vi "Process.vi"(8 "error in":errorcluster, 11 "Instrument UI.Framework-Template":refnum<class "Instrument UI.Framework-Template.lvclass">) -> (0 "error out":errorcluster, 3 "Instrument UI.Framework-Template out":refnum<class "Instrument UI.Framework-Template.lvclass">)   [LabVIEW 2019, in "Instrument UI.Framework-Template.lvclass"]
doc: "---------------------------------------------------------------\nJKI State Machine Objects™\nhttp://jki.net/state-machine-objects/\nCopyright (C) 2005-2015, JKI <info@jki.net>\nALL RIGHTS RESERVEDJKI State Machine Objects (SMO) 1.0.0.5\nJKI - JKI\nCopyright (c) 2016, JKI"
uses:
  Instrument UI.Framework-Template.lvclass
  C:/Program Files (x86)/National Instruments/LabVIEW 2019/vi.lib/JKI/JKI SMO/SMO/SMO.lvclass
  C:/Program Files (x86)/National Instruments/LabVIEW 2019/user.lib/LevyLab/Instrument Framework/Instrument UI/Instrument UI.lvclass
  C:/Program Files (x86)/National Instruments/LabVIEW 2019/vi.lib/JKI/JKI SMO/SMO.UI/SMO.UI.lvclass
  Instrument.Framework-Template/Typedefs/Instrument.Framework-Template.getAll--Cluster.ctl
  Instrument.Framework-Template/Instrument.Framework-Template.lvclass
  C:/Program Files (x86)/National Instruments/LabVIEW 2019/user.lib/LevyLab/Instrument Framework/Instrument/Instrument.lvclass
  Instrument UI.Framework-Template.UI--Cluster.ctl
  Instrument.Framework-Template/Typedefs/Instrument.Framework-Template.Configuration--Cluster.ctl
  <userlib>/LevyLab/Configuration/Configuration.lvclass
  <userlib>/LevyLab/Instrument Framework/Instrument UI/Instrument UI.lvclass/Instrument UI.ctl
  <vilib>/JKI/JKI SMO/SMO/SMO.lvclass/SMO.ctl
  <userlib>/LevyLab/Configuration/Configuration.lvclass/Configuration.ctl
  2c224a34-a253-4174-b18d-44043a318d1a.vi
  <vilib>/JKI/JKI SMO/SMO/Private/ReftoDVR--SMO.vi
  2c224a34-a253-4174-b18d-44043a318d1a.vi/26bc7fe7-399c-42c0-9e9a-60ca208975aa.vi
  2c224a34-a253-4174-b18d-44043a318d1a.vi/9995e869-8f6f-46da-9c29-74663bf4c27c.vi
  <vilib>/Utility/Data Type/Get Type Information.vi
  <vilib>/JDP Science/JSONtext/JSON text to Variant.vi
  <userlib>/LevyLab/Instrument Framework/Instrument/Instrument.lvclass
  <vilib>/JDP Science/JSONtext/LVClass Serializer/JSONtext LVClass Serializer.lvclass
  <userlib>/LevyLab/Instrument Framework/Instrument UI/Instrument UI.lvclass
  <vilib>/JKI/JKI SMO/SMO/SMO.lvclass
  <vilib>/JKI/JKI SMO/SMO.UI/SMO.UI.lvclass
  <userlib>/LevyLab/Debug/Debug.lvlib
panel:
  out "State History":string
  in  "Parameter 2":string
  out "Numeric":u32
  in  "Set Parameter":bool
  in  "Parameter":dbl
  in  "STOP":bool
  out "SMO string":string
  out "SMO Boolean":bool
  out "Logger SMO":dbl
  out "Levy 1":dbl
  # "#todo\nmake UI here. maybe include a nice picture of the hardware?"
  # "#todo\nadd buttons to do stuff (e.g., change a setting)\nButtons should trigger an event"
  # "#todo\nresize this box if you want your UI to be different size"
  # "SMO UI Template"
  # "For instructions on how to use the JKI State Machine Objects, examples and video tutorials, visit:\nhttp://jki.net/state-machine-objects/\n\nJKI State Machine Objects™\nhttp://jki.net/state-machine-objects/\nCopyright (C) 2005-2015, JKI <info@jki.net>\nALL RIGHTS RESERVED"
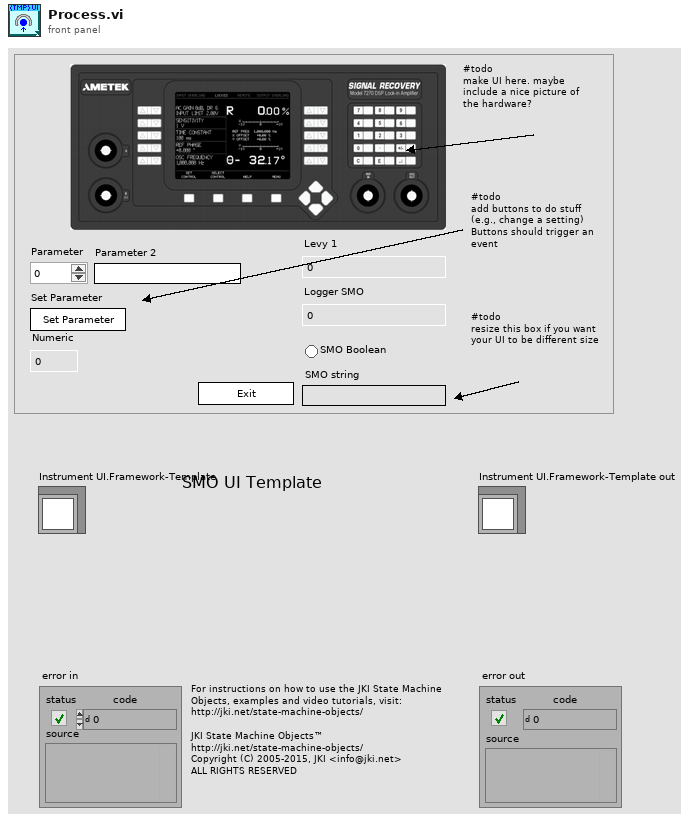
[diagram p1: front panel]
types:
  T1 = enum32{"invalid app kind", "Development System", "Run Time System", "Student Edition", "Embedded LabVIEW", "Evaluation", "Custom"}
  T2 = enum32{"Invalid", "Standard", "Closed", "Hidden", "Minimized", "Maximized"}
  T3 = typedef "Instrument.Framework-Template.lvclass/Instrument.Framework-Template.Configuration--Cluster.ctl" = cluster{"Example Setting 1":dbl, "Example Setting 2":dbl, "Example Setting 3":string}
  T4 = typedef "Instrument.Framework-Template.lvclass/Instrument.Framework-Template.getAll--Cluster.ctl" = cluster{"Levy 1":dbl, "Logger SMO":dbl, "SMO Boolean":bool, "SMO String":string}
  T5 = typedef "Instrument UI.Framework-Template.lvclass/Instrument UI.Framework-Template.UI--Cluster.ctl" = cluster{"Parameter":dbl, "Parameter 2":string}
  T6 = cluster{"Core":cluster{"Current VI Reference":refnum<vi>, "Close Panel on Exit?":bool, "Last Error":cluster{"error":errorcluster, "previous state":string, "remaining states":string}, "Shutdown?":bool}, "Instrument UI":refnum<class "Instrument UI.Framework-Template.lvclass">, "Instrument":refnum<class "Instrument.Framework-Template.lvclass">, "Configuration":refnum<class "Configuration.lvclass">, "Config Cluster":T3, "getAll":T4, "UI Cluster":T5, "UI Behavior":string, "wait":u32}
  T7 = cluster{"Current VI Reference":refnum<vi>, "Close Panel on Exit?":bool, "Last Error":cluster{"error":errorcluster, "previous state":string, "remaining states":string}, "Shutdown?":bool}
  T8 = typedef "Debug.lvlib/Attribute.Debug.lvclass/DebugBehavior.ctl" = enum16{"Normal", "Debug"}
  T9 = typedef "smo.lvlib/SMO.lvclass/Protected Events.ctl" = cluster{"StopProcesses":refnum<user-event>, "AbortProcesses":refnum<user-event>, "Config Changed":refnum<user-event>, "Dependency":refnum<user-event>}
  T10 = typedef "Instrument.lvlib/Instrument.lvclass/PublicEvents--Cluster.ctl" = cluster{"MessageFromProcess":refnum<user-event>}
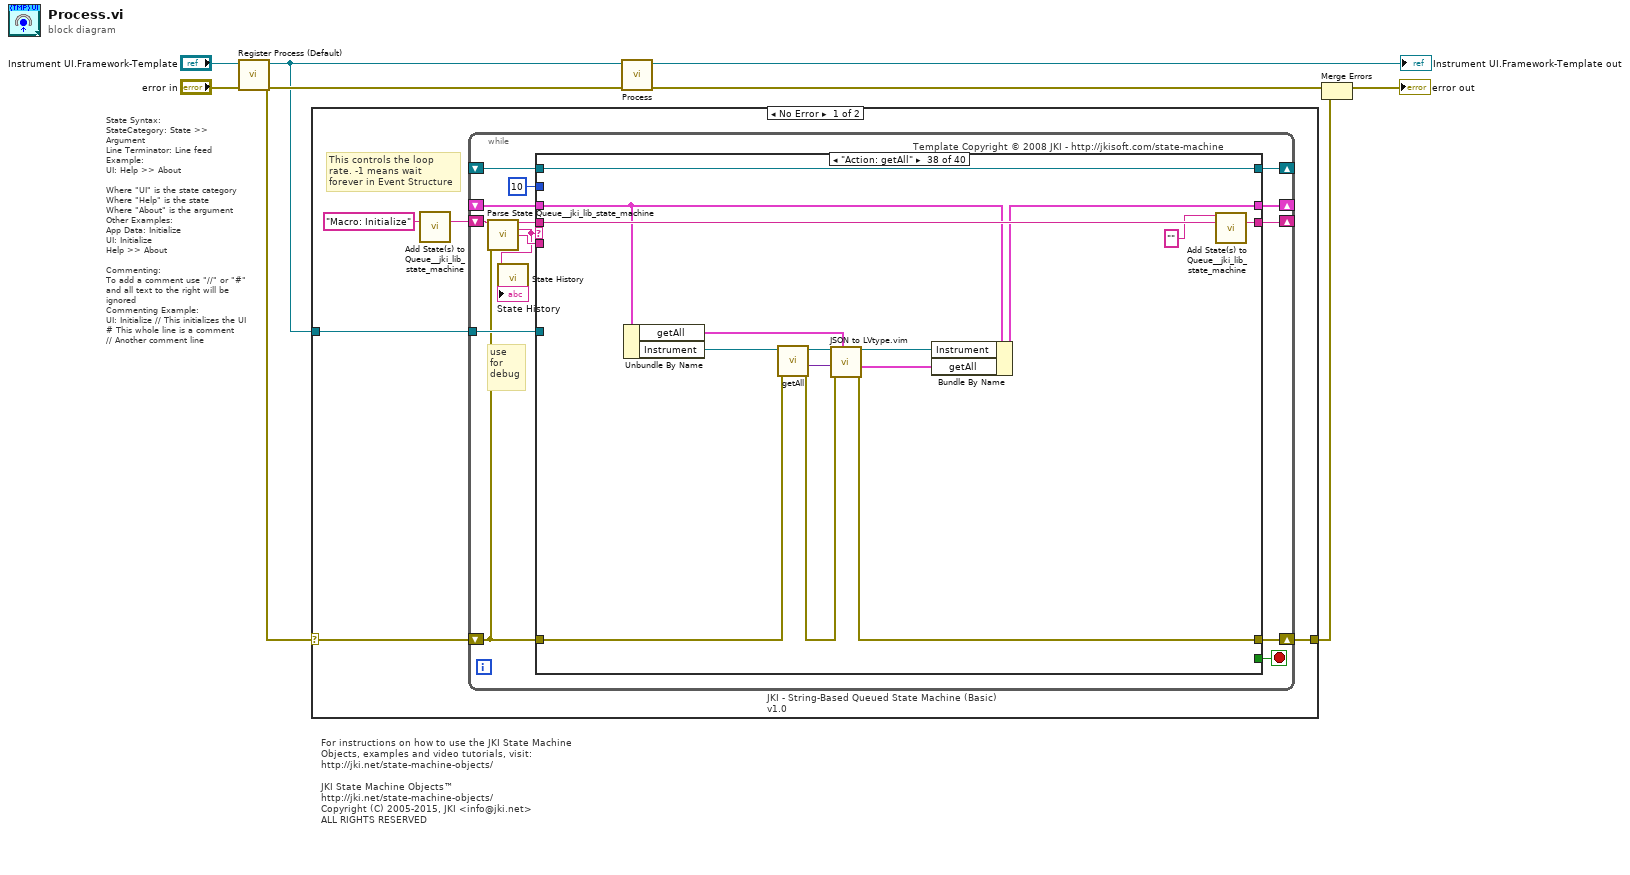
[diagram p0: block diagram]
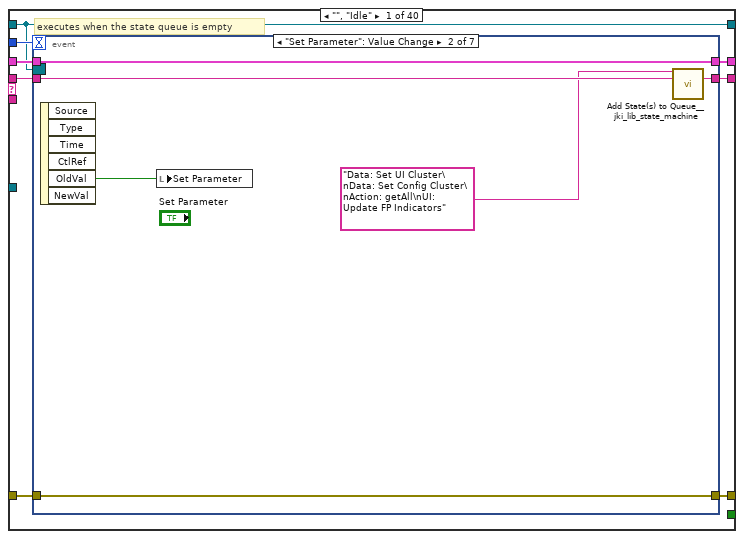
[diagram p2: hidden frame]
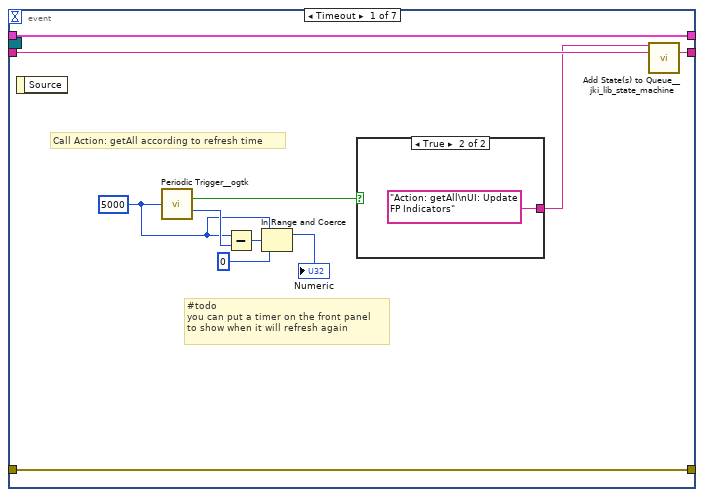
[diagram p3: hidden frame]
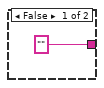
[diagram p4: hidden frame]
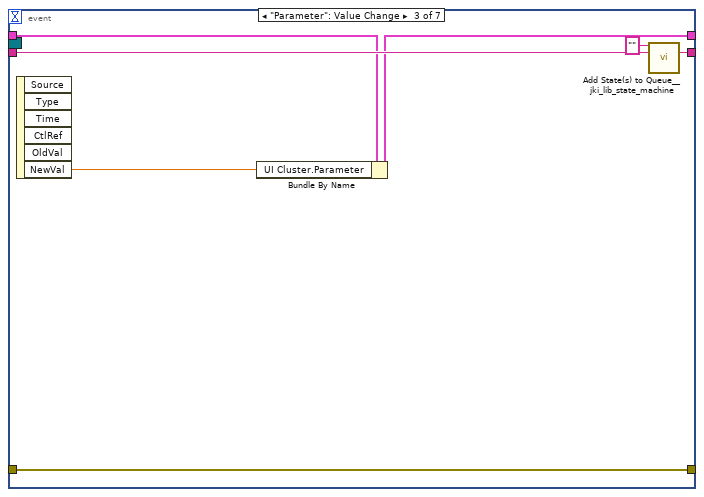
[diagram p5: hidden frame]
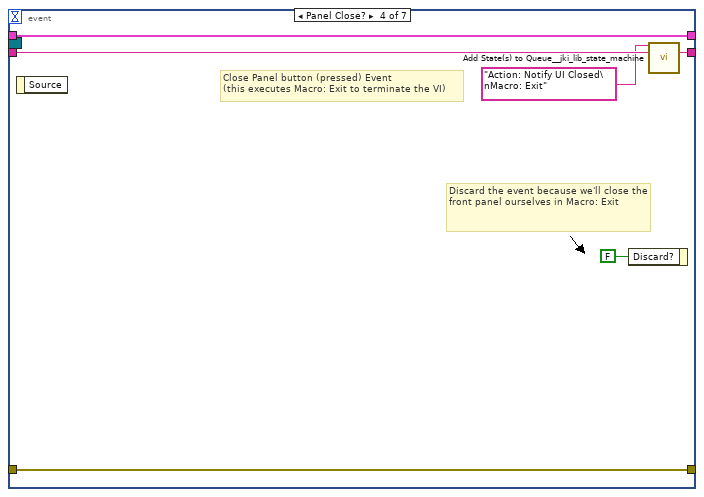
[diagram p6: hidden frame]
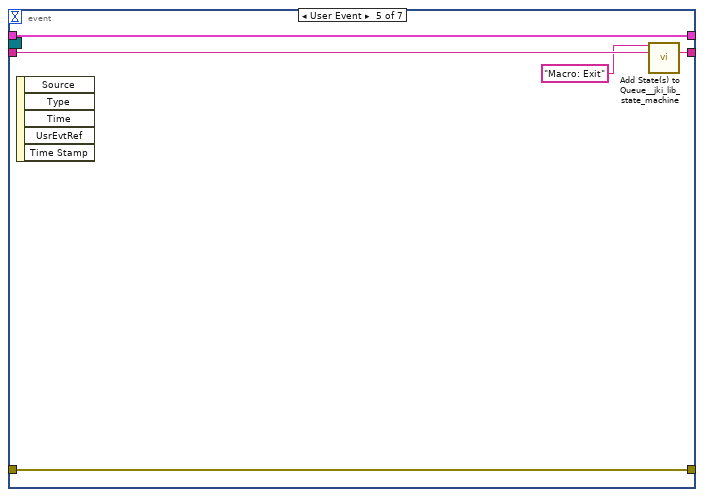
[diagram p7: hidden frame]
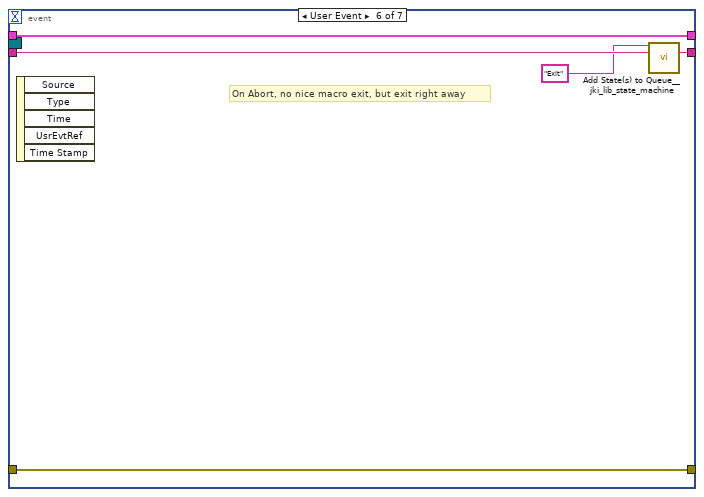
[diagram p8: hidden frame]
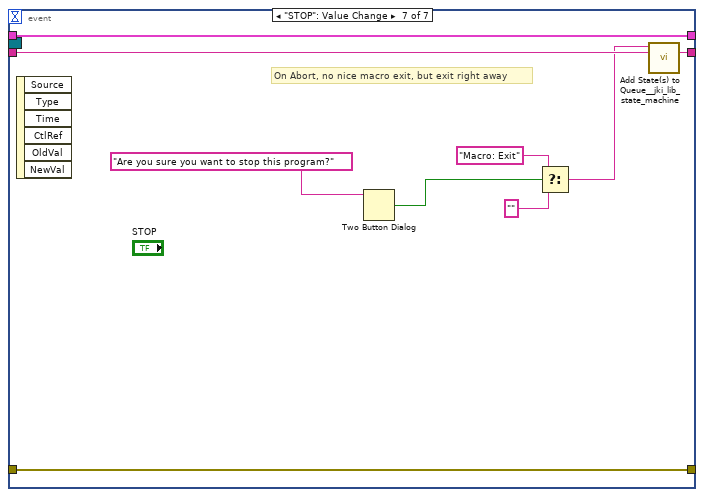
[diagram p9: hidden frame]
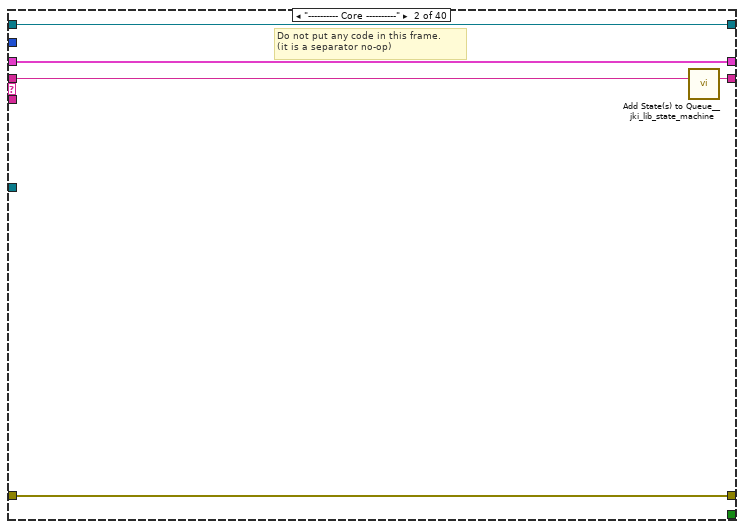
[diagram p10: hidden frame]
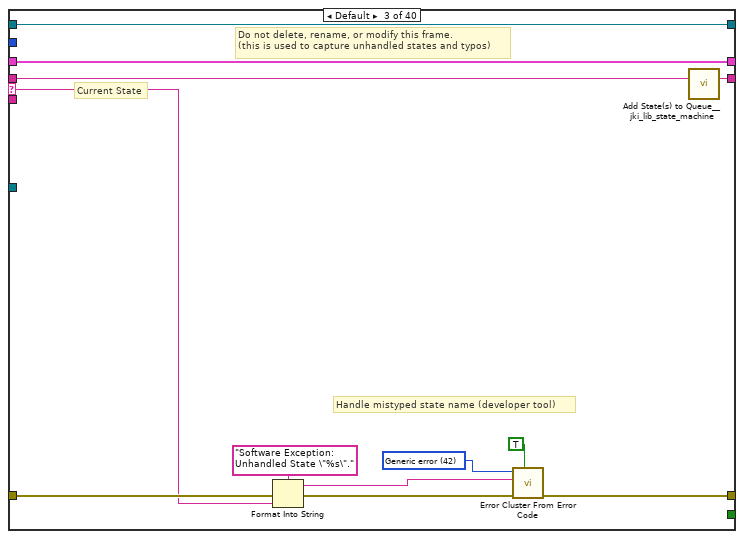
[diagram p11: hidden frame]
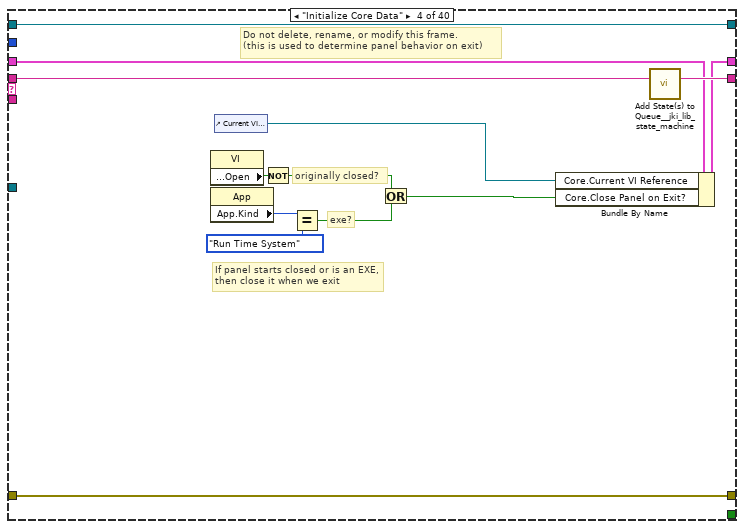
[diagram p12: hidden frame]
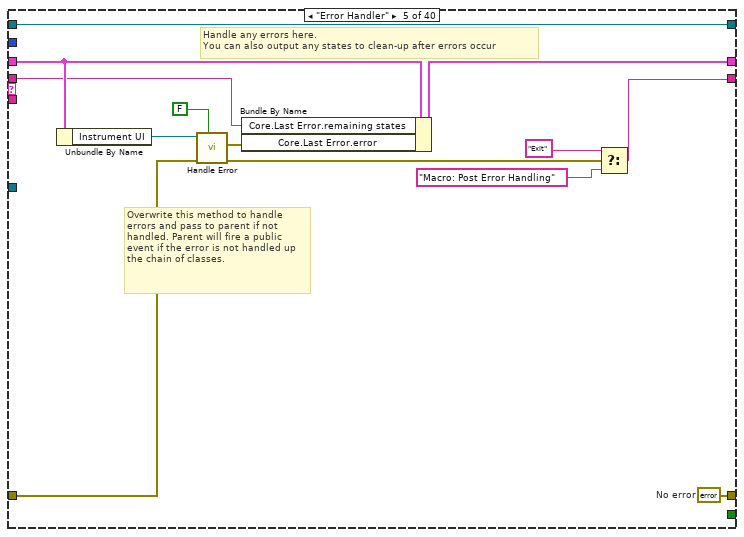
[diagram p13: hidden frame]
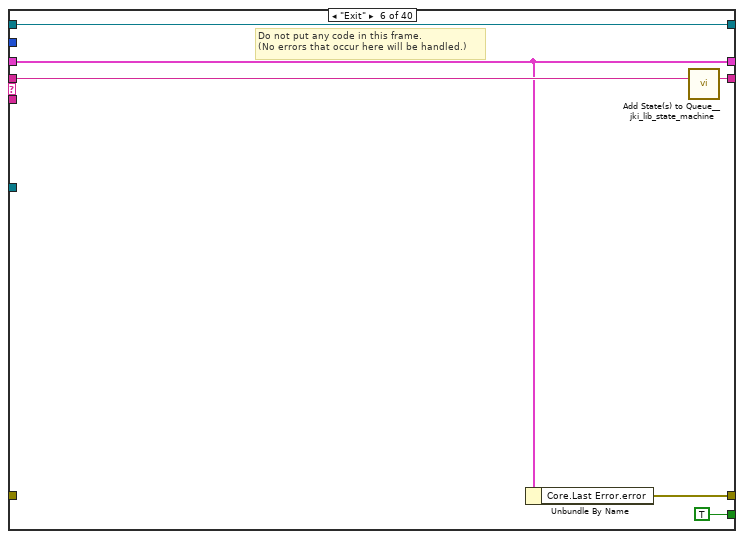
[diagram p14: hidden frame]
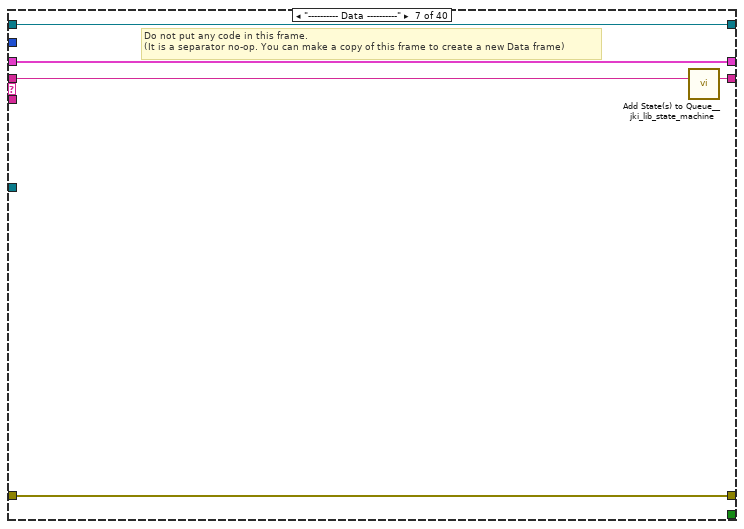
[diagram p15: hidden frame]
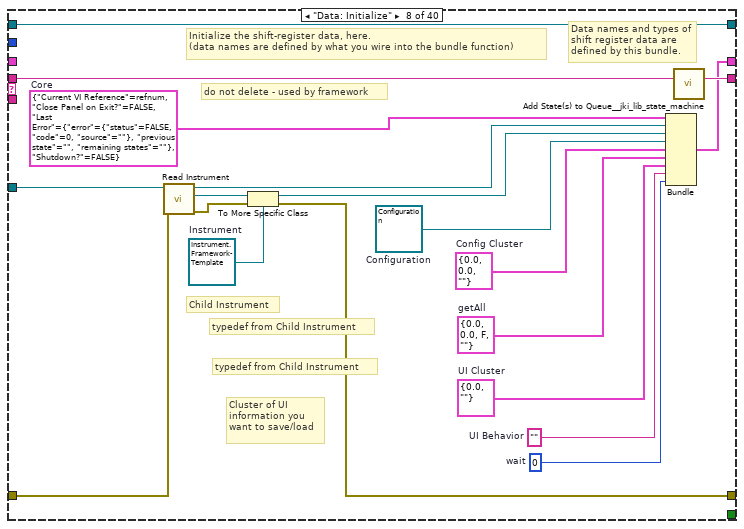
[diagram p16: hidden frame]
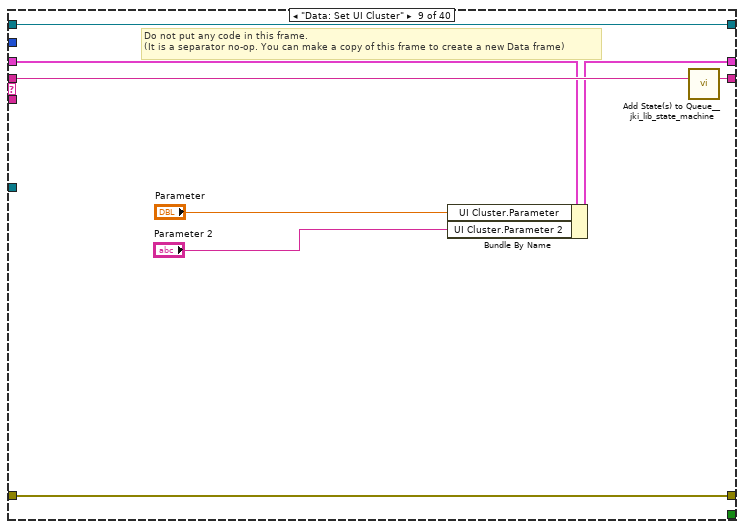
[diagram p17: hidden frame]
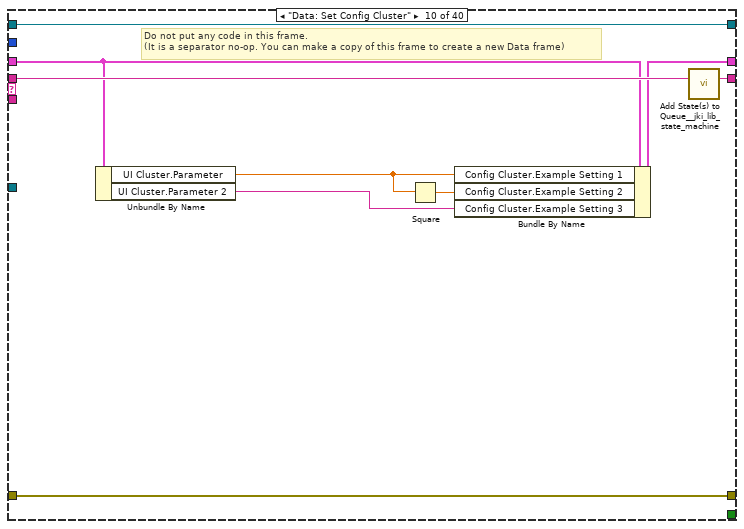
[diagram p18: hidden frame]
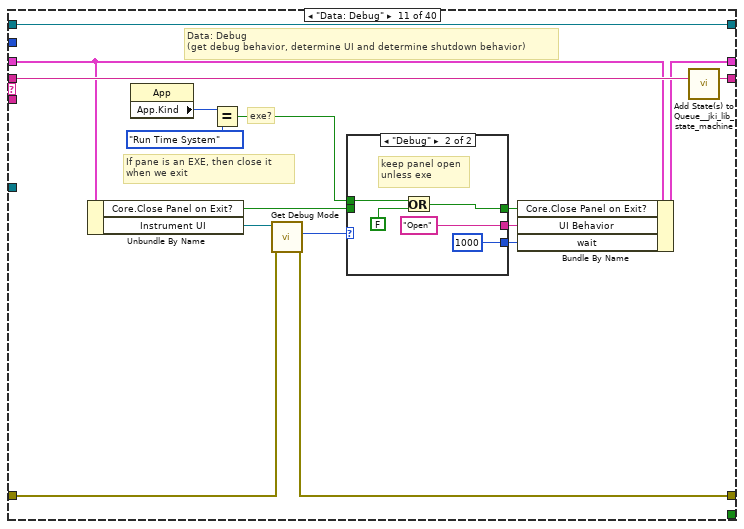
[diagram p19: hidden frame]
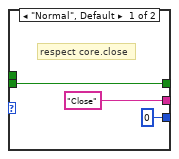
[diagram p20: hidden frame]
diagram:
  # "State Syntax:\nStateCategory: State >> Argument\nLine Terminator: Line feed\nExample:\nUI: Help >> About\n\nWhere \"UI\" is the state category\nWhere \"Help\" is the state\nWhere \"About\" is the argument\nOther Examples:\nApp Data: Initialize\nUI: Initialize\nHelp >> About\n\nCommenting:\nTo add a comment use \"//\" or \"#\" and all text to the right will be ignored\nCommenting Example:\nUI: Initialize // This initializes the UI\n# This whole line is a comment\n// Another comment line"
  # "For instructions on how to use the JKI State Machine Objects, examples and video tutorials, visit:\nhttp://jki.net/state-machine-objects/\n\nJKI State Machine Objects™\nhttp://jki.net/state-machine-objects/\nCopyright (C) 2005-2015, JKI <info@jki.net>\nALL RIGHTS RESERVED"
  n1 = call <vilib>:"Register Process (Default).vi"("error in (no error)"="error in", "SMO"="Instrument UI.Framework-Template") -> ("error out"=w5:errorcluster, "SelfRef"=w4:refnum<class "Instrument UI.Framework-Template.lvclass">)  [unwired: 8 in]
  n2 = case shown="No Error" w5 {
    selector: w5 -> [w10 w488]
    tunnel: w4 -> [w11 _]
    tunnel: [w9 w488] -> w1
    frame No Error {
      # "This controls the loop rate. -1 means wait forever in Event Structure"
      n3 = call <vilib>:"Add State(s) to Queue__jki_lib_state_machine.vi"("State(s) in (\"\")"="Macro: Initialize") -> ("States Out"=w13:string)  [unwired: 14 in]
      n4 = while "JKI - String-Based Queued State Machine (Basic) v1.0" {
        shift-right: [w22] -> _
        shift-left: _ -> [w21]
        shift-right: [w25] -> w9
        shift-left: w10 -> [w16]
        shift-right: [w24] -> _
        shift-left: w13 -> [w26]
        tunnel: w11 -> [w19]
        shift-right: [w18] -> _
        shift-left: _ -> [w17]
        stop <- w23 stop-if-true
        # "use\nfor\ndebug"
        # "Template Copyright © 2008 JKI - http://jkisoft.com/state-machine"
        n5 = call <vilib>:"Parse State Queue__jki_lib_state_machine.vi"("State Queue"=w26, "Error In (no error)"=w16) -> ("Remaining States"=w28:string, "Current State"=w15:string, "Arguments"=w27:string)  [unwired: 11 in]
        n6 = call <userlib>:"State History.vi"("Current State"=w15) -> ("State History"=→"State History":string)  [unwired: 10 in]
        n7 = case shown="\"Action: getAll\"" w15 {
          selector: w15 -> [_ _ w94 _ _ _ _ _ _ _ _ _ _ _ _ _ _ _ _ _ _ _ _ _ _ _ _ _ _ _ _ _ _ _ _ _ _ _ _ _]
          tunnel: w28 -> [w36 w92 w98 w117 w121 w136 w141 w160 w168 w177 w193 w208 w213 w220 w227 w237 w244 w260 w292 w301 w313 w323 w329 w337 w352 w357 w368 w375 w380 w393 w399 w404 w419 w427 w439 w446 w453 w467 w477 w487]
          tunnel: w27 -> [_ _ _ _ _ _ _ _ _ _ _ _ _ _ _ _ w238 w254 _ _ _ _ _ _ _ _ _ _ _ _ _ _ _ _ _ _ _ _ _ _]
          tunnel: w21 -> [w34 w89 w96 w108 w124 w132 w138 _ w164 w173 w180 w202 w210 w218 w223 w228 w242 w256 w289 w298 w303 w320 w326 w331 w341 w354 w365 w370 w377 w391 w397 w401 w412 w424 w430 w442 w447 w462 w471 w479]
          tunnel: [w33 w90 w100 w114 w126 w131 w139 w142 w166 w175 w179 w204 w211 w215 w225 w229 w239 w257 w290 w293 w311 w321 w327 w335 w350 w355 w359 w371 w378 w386 w394 w402 w405 w422 w431 w443 w448 w460 w474 w484] -> w25
          tunnel: [w35 w91 w97 w116 w118 w135 w140 w159 w167 w176 w192 w207 w212 w219 w226 w236 w243 w259 w291 w300 w312 w322 w328 w336 w351 w356 w367 w374 w379 w392 w398 w403 w418 w426 w438 w445 w452 w466 w476 w486] -> w24
          tunnel: [_ _ _ _ _ TRUE _ _ _ _ _ _ _ _ _ _ _ _ _ _ _ _ _ _ _ _ _ _ _ _ _ _ _ _ _ _ _ _ _ _] -> w23
          tunnel: [w31 w89 w96 w115 w123 w132 w138 w158 w163 w172 w181 w202 w210 w218 w223 w228 w242 w256 w289 w298 w304 w320 w326 w331 w341 w354 w365 w370 w377 w391 w397 w401 w416 w424 w428 w441 w447 w463 w472 w481] -> w22
          tunnel: 10 ("Timeout") -> [w30 _ _ _ _ _ _ _ _ _ _ _ _ _ _ _ _ _ _ _ _ _ _ _ _ _ _ _ _ _ _ _ _ _ _ _ _ _ _ _]
          tunnel: w19 -> [_ _ _ _ _ _ _ w147 _ _ _ _ _ _ _ _ _ _ _ _ _ _ _ _ _ _ _ _ _ _ _ _ _ _ _ _ _ _ _ _]
          tunnel: [w29 w88 w93 w105 w130 w133 w137 w157 w165 w174 w191 w203 w209 w217 w224 w235 w241 w253 w288 w299 w310 w319 w325 w334 w346 w353 w366 w373 w376 w390 w396 w400 w417 w425 w437 w444 w451 w465 w475 w485] -> w18
          tunnel: w17 -> [w29 w88 w93 w105 w130 w133 w137 w157 w165 w174 w191 w203 w209 w217 w224 w235 w241 w253 w288 w299 w310 w319 w325 w334 w346 w353 w366 w373 w376 _ w396 w400 w417 w425 w437 w444 w451 w465 w475 w485]
          tunnel: w16 -> [w32 w90 w99 w114 w120 _ w139 w146 w166 w175 w178 w205 w211 w216 w225 w229 w240 w258 w290 w293 w311 w321 w327 w335 w350 w355 w360 w372 w378 w388 w395 w402 w414 w420 w432 w443 w449 w454 w468 w480]
          frame "", "Idle" {
            # "executes when the state queue is empty"
            n8 = event shown="[1] \"Set Parameter\": Value Change" {
              selector: w29 -> [_ _ _ _ _ _ _]
              dyn-events: _ -> [_ _ _ _ _ _ _]
              timeout: w30 -> [_ _ _ _ _ _ _]
              tunnel: w36 -> [w47 w55 w62 w68 w73 w78 w87]
              tunnel: [w46 w54 w61 w67 w72 w77 w86] -> w35
              tunnel: w34 -> [w44 w52 w58 w64 w70 w75 w84]
              tunnel: [w45 w53 w60 w63 w71 w76 w85] -> w33
              tunnel: w32 -> [w45 w53 w60 w63 w71 w76 w85]
              tunnel: [w44 w52 w57 w64 w70 w75 w84] -> w31
              event Timeout {
                w38 = u32 5000 ("time (ms)")
                # "#todo\nyou can put a timer on the front panel\nto show when it will refresh again"
                # "Call Action: getAll according to refresh time"
                n9 = event-data() -> ()  [unwired: 1 in, 1 out]
                n10 = call <userlib>:"Periodic Trigger__ogtk.vi"("time (ms)"=w38) -> ("Triggered"=w42:bool, "timer value"=w41:u32)  [unwired: 12 in, 1 out]
                n11 = Subtract(x=w38, y=w41) -> (x-y=w40:u32)
                n12 = In Range and Coerce(upper limit=w38, x=w40, lower limit=u32 0) -> (coerced(x)=→"Numeric":u32)  [unwired: 1 out]
                n13 = case shown="True" w42 {
                  tunnel: ["" ("State(s) in Front (\"\")") "Action: getAll\nUI: Update FP Indicators" ("State(s) in Front (\"\")")] -> w43
                  frame False {
                  }
                  frame True {
                  }
                }
                n14 = call <vilib>:"Add State(s) to Queue__jki_lib_state_machine.vi"("State(s) in Front (\"\")"=w43, "State(s) in (\"\")"=w47) -> ("States Out"=w46:string)  [unwired: 13 in]
              }
              event "Set Parameter": Value Change {
                n15 = event-data() -> ("OldVal"=w51:bool)  [unwired: 1 in, 5 out]
                n16 = local write "Set Parameter"(w51) -> ()
                n17 = call <vilib>:"Add State(s) to Queue__jki_lib_state_machine.vi"("State(s) in Front (\"\")"="Data: Set UI Cluster\nData: Set Config Cluster\nAction: getAll\nUI: Update FP Indicators" ("State(s) in Front (\"\")"), "State(s) in (\"\")"=w55) -> ("States Out"=w54:string)  [unwired: 13 in]
              }
              event "Parameter": Value Change {
                n18 = event-data() -> ("NewVal"=w59:dbl)  [unwired: 1 in, 5 out]
                n19 = Bundle By Name(cluster=w58, "UI Cluster.Parameter"=w59) -> (w57:T6)
                n20 = call <vilib>:"Add State(s) to Queue__jki_lib_state_machine.vi"("State(s) in Front (\"\")"="" ("State(s) in Front (\"\")"), "State(s) in (\"\")"=w62) -> ("States Out"=w61:string)  [unwired: 13 in]
              }
              event Panel Close? {
                # "Discard the event because we'll close the front panel ourselves in Macro: Exit"
                # "Close Panel button (pressed) Event\n(this executes Macro: Exit to terminate the VI)"
                n21 = event-data() -> ()  [unwired: 1 in, 1 out]
                n22 = event-data("Discard?"=FALSE) -> ()  [unwired: 1 in, 1 out]
                n23 = call <vilib>:"Add State(s) to Queue__jki_lib_state_machine.vi"("State(s) in Front (\"\")"="Action: Notify UI Closed\nMacro: Exit", "State(s) in (\"\")"=w68) -> ("States Out"=w67:string)  [unwired: 13 in]
              }
              event User Event {
                n24 = event-data() -> ()  [unwired: 1 in, 5 out]
                n25 = call <vilib>:"Add State(s) to Queue__jki_lib_state_machine.vi"("State(s) in Front (\"\")"="Macro: Exit", "State(s) in (\"\")"=w73) -> ("States Out"=w72:string)  [unwired: 13 in]
              }
              event User Event {
                # "On Abort, no nice macro exit, but exit right away"
                n26 = event-data() -> ()  [unwired: 1 in, 5 out]
                n27 = call <vilib>:"Add State(s) to Queue__jki_lib_state_machine.vi"("State(s) in Front (\"\")"="Exit", "State(s) in (\"\")"=w78) -> ("States Out"=w77:string)  [unwired: 13 in]
              }
              event "STOP": Value Change {
                # "On Abort, no nice macro exit, but exit right away"
                n28 = event-data() -> ()  [unwired: 1 in, 6 out]
                n29 = Two Button Dialog(message="Are you sure you want to stop this program?") -> (T button?=w83:bool)  [unwired: 2 in]
                n30 = Select(t="Macro: Exit", s=w83, f="") -> (s? t:f=w79:string)
                n31 = call <vilib>:"Add State(s) to Queue__jki_lib_state_machine.vi"("State(s) in Front (\"\")"=w79, "State(s) in (\"\")"=w87) -> ("States Out"=w86:string)  [unwired: 13 in]
              }
            }
          }
          frame "---------- Core ----------" {
            # "Do not put any code in this frame.\n(it is a separator no-op)"
            n32 = call <vilib>:"Add State(s) to Queue__jki_lib_state_machine.vi"("State(s) in (\"\")"=w92) -> ("States Out"=w91:string)  [unwired: 14 in]
          }
          frame Default {
            w103 = 42 items=["No error", "Argument error", "Memory is full", "Out of zone", "End of file", "File already open", "Generic file I/O error", "File not found", "File permission error", "Disk is full", "Duplicate path", "Too many files open", "System feature not enabled", "Resource file not found", "Cannot add resource", "Resource not found", "Image not found", "Image memory error", "Pen does not exist", "Config type invalid", "Config token not found", "Config parse error", "Config memory error", "Bad external code format", "Bad external code offset", "External code not present", "Null window", "Destroy window error", "Null menu", "Print aborted", "Bad print record", "Print driver error", "Windows error during printing", "Memory error during printing", "Print dialog error", "Generic print error", "Invalid device refnum", "Device not found", "Device parameter error", "Device unit error", "Cannot open device", "Device call aborted", "Generic error", "Cancelled by user", "Object ID too low", "Object ID too high", "Object not in heap", "Unknown heap", "Unknown object (invalid DefProc)", "Unknown object (DefProc not in table)", "Message out of range", "Invalid (null) method", "Unknown message", "Manager call not supported", "Bad address", "Network operation in progress", "Network operation timed out", "Connection is busy", "Network attribute not supported", "Network error", "Address in use", "System out of memory", "Connection aborted", "Connection refused", "Not connected", "Already connected", "Connection closed", "Initialization error (interapplication manager)", "Bad occurrence", "Wait on unbound occurrence handler", "Occurrence queue overflow", "Datalog type conflict", "Unused", "Unrecognized type (interapplication manager)", "Memory corrupt", "Failed to make temporary DLL", "Old CIN version", "Drag socket not found", "Failed to load drop-object", "Failed to register OLE object", "Failed to release OLE object", "Format specifier type mismatch", "Unknown format specifier", "Too few format specifiers", "Too many format specifiers", "Scan failed", "Newer CIN version", "Error converting to variant", "Runtime menu error", "Password tampered", "Variant attribute not found", "Incompatible variant data type", "Event data is not available", "Event Store is not present", "Occurrence is not found", "Event Queue is not created", "Event info is not available", "Refnum passed is NULL", "Error retrieving Class GUID", "Error retrieving CoClass GUID", "Error retrieving TypeLib GUID.", "Bad built application magic bytes.", "Specific driver is different from the specific driver associated with the Logical Name.", "There is no session opened to the class driver.", "Max Error", "MAX - Error with config objects", "MAX - Error loading configuration", "MAX - Group not supported"]
            # "Current State"
            # "Do not delete, rename, or modify this frame.\n(this is used to capture unhandled states and typos)"
            # "Handle mistyped state name (developer tool)"
            n33 = Format Into String(format string="Software Exception: Unhandled State \"%s\"." ("message"), error in=w99, w94) -> (resulting string=w102:string, error out=w101:errorcluster)  [unwired: 1 in]
            n34 = call <vilib>:"Error Cluster From Error Code.vi"("show call chain? (False)"=TRUE, "error in (no error)"=w101, "error message (\"\")"=w102, "error code (0)"=w103) -> ("error out"=w100:errorcluster)  [unwired: 5 in]
            n35 = call <vilib>:"Add State(s) to Queue__jki_lib_state_machine.vi"("State(s) in (\"\")"=w98) -> ("States Out"=w97:string)  [unwired: 14 in]
          }
          frame "Initialize Core Data" {
            # "Do not delete, rename, or modify this frame.\n(this is used to determine panel behavior on exit)"
            # "originally closed?"
            # "exe?"
            # "If panel starts closed or is an EXE, then close it when we exit"
            n36 = property class="VI"() -> ("Front Panel.Open"=w113:bool)  [unwired: 2 in, 2 out]
            n37 = property class="App"() -> ("App.Kind"=w112:T1)  [unwired: 2 in, 2 out]
            n38 = control-ref of="Current VI Reference"() -> (w106:refnum<vi>)
            n39 = Not(x=w113) -> (.not. x?=w110:bool)
            n40 = Equal?(x=w112, y=T1."Run Time System" ("Application:Kind")) -> (x = y?=w109:bool)
            n41 = Or(x=w110, y=w109) -> (x .or. y?=w107:bool)
            n42 = Bundle By Name(cluster=w108, "Core.Current VI Reference"=w106, "Core.Close Panel on Exit?"=w107) -> (w115:T6)
            n43 = call <vilib>:"Add State(s) to Queue__jki_lib_state_machine.vi"("State(s) in (\"\")"=w117) -> ("States Out"=w116:string)  [unwired: 14 in]
          }
          frame "Error Handler" {
            w126 = errorcluster {"status"=FALSE, "code"=0, "source"=""}  # No error
            # "Overwrite this method to handle errors and pass to parent if not handled. Parent will fire a public event if the error is not handled up the chain of classes."
            # "Handle any errors here.\nYou can also output any states to clean-up after errors occur"
            n44 = Unbundle By Name(w124) -> ("Instrument UI"=w129:refnum<class "Instrument UI.Framework-Template.lvclass">)
            n45 = call-dynamic "Handle Error.vi"("Stop on Unhandled Error (T)"=FALSE, "error in"=w120, "SMO"=w129) -> ("handling error"=w127:errorcluster, "Unhandled error"=w125:errorcluster)  [unwired: 6 in, 1 out]
            n46 = Bundle By Name(cluster=w124, "Core.Last Error.remaining states"=w121, "Core.Last Error.error"=w125) -> (w123:T6)
            n47 = Select(t="Exit", s=w127, f="Macro: Post Error Handling") -> (s? t:f=w118:string)
          }
          frame "Exit" {
            # "Do not put any code in this frame.\n(No errors that occur here will be handled.)"
            n48 = Unbundle By Name(w132) -> ("Core.Last Error.error"=w131:errorcluster)
            n49 = call <vilib>:"Add State(s) to Queue__jki_lib_state_machine.vi"("State(s) in (\"\")"=w136) -> ("States Out"=w135:string)  [unwired: 14 in]
          }
          frame "---------- Data ----------" {
            # "Do not put any code in this frame.\n(It is a separator no-op. You can make a copy of this frame to create a new Data frame)"
            n50 = call <vilib>:"Add State(s) to Queue__jki_lib_state_machine.vi"("State(s) in (\"\")"=w141) -> ("States Out"=w140:string)  [unwired: 14 in]
          }
          frame "Data: Initialize" {
            w143 = u32 0  # wait
            w144 = ""  # UI Behavior
            w148 = refnum<class "Configuration.lvclass"> refnum  # Configuration
            w150 = T3 {"Example Setting 1"=0.0, "Example Setting 2"=0.0, "Example Setting 3"=""}  # Config Cluster
            w152 = T5 {"Parameter"=0.0, "Parameter 2"=""}  # UI Cluster
            w154 = refnum<class "Instrument.Framework-Template.lvclass"> refnum  # Instrument
            w155 = T4 {"Levy 1"=0.0, "Logger SMO"=0.0, "SMO Boolean"=FALSE, "SMO String"=""}  # getAll
            w156 = T7 {"Current VI Reference"=refnum, "Close Panel on Exit?"=FALSE, "Last Error"={"error"={"status"=FALSE, "code"=0, "source"=""}, "previous state"="", "remaining states"=""}, "Shutdown?"=FALSE}  # Core
            # "typedef from Child Instrument"
            # "Cluster of UI\ninformation you\nwant to save/load"
            # "Child Instrument"
            # "typedef from Child Instrument"
            # "do not delete - used by framework"
            # "Data names and types of shift register data are defined by this bundle."
            # "Initialize the shift-register data, here.\n(data names are defined by what you wire into the bundle function)"
            n51 = call <userlib>:"Read Instrument.vi"("error in (no error)"=w146, "Instrument UI in"=w147) -> ("error out"=w151:errorcluster, "Instrument"=w153:refnum<class "Instrument.lvclass">, "Instrument UI"=w145:refnum<class "Instrument UI.Framework-Template.lvclass">)  [unwired: 7 in]
            n52 = To More Specific Class(target class=w154, reference=w153, error in=w151) -> (specific class reference=w149:refnum<class "Instrument.Framework-Template.lvclass">, error out=w142:errorcluster)
            n53 = Bundle("Core"=w156, "Instrument UI"=w145, "Instrument"=w149, "Configuration"=w148, "Config Cluster"=w150, "getAll"=w155, "UI Cluster"=w152, "UI Behavior"=w144, "wait"=w143) -> (w158:T6)  [unwired: 1 in]
            n54 = call <vilib>:"Add State(s) to Queue__jki_lib_state_machine.vi"("State(s) in (\"\")"=w160) -> ("States Out"=w159:string)  [unwired: 14 in]
          }
          frame "Data: Set UI Cluster" {
            # "Do not put any code in this frame.\n(It is a separator no-op. You can make a copy of this frame to create a new Data frame)"
            n55 = Bundle By Name(cluster=w164, "UI Cluster.Parameter"="Parameter", "UI Cluster.Parameter 2"="Parameter 2") -> (w163:T6)
            n56 = call <vilib>:"Add State(s) to Queue__jki_lib_state_machine.vi"("State(s) in (\"\")"=w168) -> ("States Out"=w167:string)  [unwired: 14 in]
          }
          frame "Data: Set Config Cluster" {
            # "Do not put any code in this frame.\n(It is a separator no-op. You can make a copy of this frame to create a new Data frame)"
            n57 = Unbundle By Name(w173) -> ("UI Cluster.Parameter"=w170:dbl, "UI Cluster.Parameter 2"=w171:string)
            n58 = Square(x=w170) -> (x^2=w169:dbl)
            n59 = Bundle By Name(cluster=w173, "Config Cluster.Example Setting 1"=w170, "Config Cluster.Example Setting 2"=w169, "Config Cluster.Example Setting 3"=w171) -> (w172:T6)
            n60 = call <vilib>:"Add State(s) to Queue__jki_lib_state_machine.vi"("State(s) in (\"\")"=w177) -> ("States Out"=w176:string)  [unwired: 14 in]
          }
          frame "Data: Debug" {
            # "exe?"
            # "If pane is an EXE, then close it when we exit"
            # "Data: Debug\n(get debug behavior, determine UI and determine shutdown behavior)"
            n61 = Unbundle By Name(w180) -> ("Core.Close Panel on Exit?"=w183:bool, "Instrument UI"=w190:refnum<class "Instrument UI.Framework-Template.lvclass">)
            n62 = property class="App"() -> ("App.Kind"=w186:T1)  [unwired: 2 in, 2 out]
            n63 = Equal?(x=w186, y=T1."Run Time System" ("Application:Kind")) -> (x = y?=w182:bool)
            n64 = call <userlib>:"Get Debug Mode.vi"("error in (no error)"=w178, "SMO"=w190) -> ("error out"=w179:errorcluster, "Behavior"=w189:T8)  [unwired: 7 in, 1 out]
            n65 = case shown="\"Debug\"" w189 {
              tunnel: ["Close" "Open"] -> w188
              tunnel: [u32 0 ("wait") u32 1000 ("wait")] -> w187
              tunnel: [w194 w197] -> w184
              tunnel: w183 -> [w194 _]
              tunnel: w182 -> [_ w199]
              frame "Normal", Default {
                # "respect core.close"
              }
              frame "Debug" {
                # "keep panel open\nunless exe"
                n66 = Or(x=w199, y=FALSE) -> (x .or. y?=w197:bool)
              }
            }
            n67 = Bundle By Name(cluster=w180, "Core.Close Panel on Exit?"=w184, "UI Behavior"=w188, "wait"=w187) -> (w181:T6)
            n68 = call <vilib>:"Add State(s) to Queue__jki_lib_state_machine.vi"("State(s) in (\"\")"=w193) -> ("States Out"=w192:string)  [unwired: 14 in]
          }
          frame "Data: Cleanup" {
            # "Cleanup any data and references, here.\n(this is called automatically, by the Macro: Exit)"
            n69 = Unbundle By Name(w202) -> ("Core.Current VI Reference"=w206:refnum<vi>)
            n70 = Close Reference(reference=w206, error in (no error)=w205) -> (error out=w204:errorcluster)
            n71 = call <vilib>:"Add State(s) to Queue__jki_lib_state_machine.vi"("State(s) in (\"\")"=w208) -> ("States Out"=w207:string)  [unwired: 14 in]
          }
          frame "---------- UI ----------" {
            # "Do not put any code in this frame.\n(It is a separator no-op. You can make a copy of this frame to create a new UI frame)"
            n72 = call <vilib>:"Add State(s) to Queue__jki_lib_state_machine.vi"("State(s) in (\"\")"=w213) -> ("States Out"=w212:string)  [unwired: 14 in]
          }
          frame "UI: Initialize" {
            # "size window to decoration box on front panel"
            # "Initialize the User Interface, here.\n(this is called automatically, by the Macro: Init)"
            n73 = invoke on="STOP" class="Bool (strict)" method="Reinit To Default"() -> ()  [unwired: 3 in, 3 out]
            n74 = call <userlib>:"Fit VI window to Largest Dec__ogtk.vi"("error in (no error)"=w216, "border spacing (2 px)"=0) -> ("error out"=w215:errorcluster)  [unwired: 4 in, 1 out]
            n75 = call <vilib>:"Add State(s) to Queue__jki_lib_state_machine.vi"("State(s) in (\"\")"=w220) -> ("States Out"=w219:string)  [unwired: 14 in]
          }
          frame "UI: Update FP Controls" {
            # "Do not put any code in this frame.\n(It is a separator no-op. You can make a copy of this frame to create a new UI frame)"
            n76 = Unbundle By Name(w223) -> ("UI Cluster.Parameter"=w221:dbl, "UI Cluster.Parameter 2"=w222:string)
            n77 = local write "Parameter 2"(w222) -> ()
            n78 = local write "Parameter"(w221) -> ()
            n79 = call <vilib>:"Add State(s) to Queue__jki_lib_state_machine.vi"("State(s) in (\"\")"=w227) -> ("States Out"=w226:string)  [unwired: 14 in]
          }
          frame "UI: Update FP Indicators" {
            # "do this way to have nicer UI or only display what you want"
            n80 = Unbundle By Name(w228) -> ("getAll"=w230:T4)
            n81 = Unbundle By Name(w230) -> ("Levy 1"=→"Levy 1":dbl, "Logger SMO"=→"Logger SMO":dbl, "SMO Boolean"=→"SMO Boolean":bool, "SMO String"=→"SMO string":string)
            n82 = call <vilib>:"Add State(s) to Queue__jki_lib_state_machine.vi"("State(s) in (\"\")"=w237) -> ("States Out"=w236:string)  [unwired: 14 in]
          }
          frame "UI: Cursor Set" {
            # "Argument"
            # "Initialize the User Interface, here.\n(this is called automatically, by the Macro: Init)"
            n83 = disable-structure shown="Default" {
              disable-tunnel: w240 -> [w245 w248]
              disable-tunnel: [w245 w247] -> w239
              disable-tunnel: w238 -> [_ w246]
              frame condition #0 {
              }
              frame condition #1 (active) {
                n84 = case shown="\"Busy\"" w246 {
                  tunnel: w248 -> [w250 w252]
                  tunnel: [w249 w251] -> w247
                  frame "Idle", Default {
                    n85 = call <vilib>:"Unset Busy.vi"("error in (no error)"=w250) -> ("error out"=w249:errorcluster)  [unwired: 10 in]
                  }
                  frame "Busy" {
                    n86 = call <vilib>:"Set Busy.vi"("error in (no error)"=w252) -> ("error out"=w251:errorcluster)  [unwired: 9 in, 1 out]
                  }
                }
              }
            }
            n87 = call <vilib>:"Add State(s) to Queue__jki_lib_state_machine.vi"("State(s) in (\"\")"=w244) -> ("States Out"=w243:string)  [unwired: 14 in]
          }
          frame "UI: Front Panel State" {
            # "Argument"
            # "Set Front Panel Open or Closed\n(Usage: \"UI: Front Panel State >> Open|Close\")"
            n88 = Unbundle By Name(w256) -> ("Core.Current VI Reference"=w255:refnum<vi>)
            n89 = disable-structure shown="Default" {
              disable-tunnel: w258 -> [w264 w287]
              disable-tunnel: [w263 w287] -> w257
              disable-tunnel: w255 -> [w262 _]
              disable-tunnel: w254 -> [w261 _]
              frame condition #0 (active) {
                n90 = case shown="\"Close\"" w261 {
                  tunnel: w264 -> [w268 w281]
                  tunnel: [w270 w282] -> w263
                  tunnel: w262 -> [w269 w279]
                  frame "Open", Default {
                    n91 = property class="VI"(reference=w269, error in=w268) -> (reference out=w266:refnum<vi>, error out=w267:errorcluster, "FP.State"=w265:T2)
                    n92 = case shown="\"Closed\"" w265 {
                      tunnel: [w273 w276] -> w270
                      tunnel: w267 -> [w272 w276]
                      tunnel: w266 -> [w271 _]
                      frame "Closed" {
                        n93 = invoke class="VI" method="FP.Open"(reference=w271, error in=w272, "Activate"=TRUE, "State"=T2."Standard") -> (error out=w273:errorcluster)  [unwired: 1 in, 4 out]
                      }
                      frame Default {
                      }
                    }
                  }
                  frame "Close" {
                    n94 = property class="VI"(reference=w279, error in=w281) -> (reference out=w278:refnum<vi>, error out=w280:errorcluster, "FP.State"=w277:T2)
                    n95 = case shown="Default" w277 {
                      tunnel: [w283 w286] -> w282
                      tunnel: w280 -> [w283 w285]
                      tunnel: w278 -> [_ w284]
                      frame "Invalid", "Closed" {
                      }
                      frame Default {
                        n96 = invoke class="VI" method="FP.Close"(reference=w284, error in=w285) -> (error out=w286:errorcluster)  [unwired: 1 in, 2 out]
                      }
                    }
                  }
                }
              }
              frame condition #1 {
              }
            }
            n97 = call <vilib>:"Add State(s) to Queue__jki_lib_state_machine.vi"("State(s) in (\"\")"=w260) -> ("States Out"=w259:string)  [unwired: 14 in]
          }
          frame "---------- Macro ----------" {
            # "Do not put any code in this frame.\n(It is a separator no-op. You can make a copy of this frame to create a new Macro frame)"
            n98 = call <vilib>:"Add State(s) to Queue__jki_lib_state_machine.vi"("State(s) in (\"\")"=w292) -> ("States Out"=w291:string)  [unwired: 14 in]
          }
          frame "Macro: Initialize" {
            w294 = "UI: Initialize\nMacro: Read UI Config\nAction: Open\nUI: Front Panel State >> Close\nMacro: Debug"  # UI: Initialize Macro: Read UI Config Action: Open UI: Front Panel State >> Close Macro: Debug
            # "Initialization Macro\n(This is called once, when the VI starts)"
            n99 = call <vilib>:"Add State(s) to Queue__jki_lib_state_machine.vi"("State(s) in Front (\"\")"="Data: Initialize\nInitialize Core Data\nEvents: Register", "State(s) in (\"\")"="Process: Sync", "State(s) at Back (\"\")"=w294) -> ("States Out"=w296:string)  [unwired: 12 in]
            n100 = call <vilib>:"Add State(s) to Queue__jki_lib_state_machine.vi"("State(s) in Front (\"\")"=w296, "State(s) in (\"\")"=w301) -> ("States Out"=w300:string)  [unwired: 13 in]
          }
          frame "Macro: Post Error Handling" {
            # "Clear Last Error?"
            n101 = Unbundle By Name(w303) -> ("Core.Last Error.remaining states"=w305:string, "Core.Shutdown?"=w306:bool)
            n102 = Unbundle By Name(w303) -> ("Core.Last Error.error"=w309:errorcluster)
            n103 = case shown="False" FALSE {
              tunnel: w309 -> [w317 _]
              tunnel: [w317 _] -> w308
              frame False {
              }
              frame True {
              }
            }
            n104 = case shown="False" w306 {
              tunnel: w305 -> [w314 w316]
              tunnel: [w314 w315] -> w302
              frame False {
                # "These are the remaining states (at the moment the error occured). States can be altered according to business logic."
                # "NOT SHUTTING DOWN"
              }
              frame True {
                # "Developer can decide to alter the states but should be aware that during the shutdown process, there are certain states that must be run for the SMO to properly shut itself (and this process) down. As such, one can add states to perform additional clean-ups, but should append the remaining state to be executed."
                # "SHUTTING DOWN"
                n105 = call <vilib>:"Add State(s) to Queue__jki_lib_state_machine.vi"("State(s) in (\"\")"=w316) -> ("States Out"=w315:string)  [unwired: 14 in]
              }
            }
            n106 = Bundle By Name(cluster=w303, "Core.Last Error.error"=w308) -> (w304:T6)
            n107 = call <vilib>:"Add State(s) to Queue__jki_lib_state_machine.vi"("State(s) in Front (\"\")"=w302, "State(s) in (\"\")"=w313) -> ("States Out"=w312:string)  [unwired: 13 in]
          }
          frame "Macro: Read UI Config" {
            # "Do not put any code in this frame.\n(It is a separator no-op. You can make a copy of this frame to create a new Macro frame)"
            n108 = call <vilib>:"Add State(s) to Queue__jki_lib_state_machine.vi"("State(s) in Front (\"\")"="Configuration: Initialize\nConfiguration: Read UI Config File\nUI: Update FP Controls" ("State(s) in Front (\"\")"), "State(s) in (\"\")"=w323) -> ("States Out"=w322:string)  [unwired: 13 in]
          }
          frame "Macro: Write UI Config" {
            # "Do not put any code in this frame.\n(It is a separator no-op. You can make a copy of this frame to create a new Macro frame)"
            n109 = call <vilib>:"Add State(s) to Queue__jki_lib_state_machine.vi"("State(s) in Front (\"\")"="Data: Set UI Cluster\nConfiguration: Write UI Config File" ("State(s) in Front (\"\")"), "State(s) in (\"\")"=w329) -> ("States Out"=w328:string)  [unwired: 13 in]
          }
          frame "Macro: Debug" {
            n110 = Unbundle By Name(w331) -> ("UI Behavior"=w333:string)
            n111 = Format Into String(format string="Data: Debug\nUI: Front Panel State >> %s\n//UI: Wait" ("State(s) in Front (\"\")"), w333) -> (resulting string=w330:string)  [unwired: 2 in, 1 out]
            n112 = call <vilib>:"Add State(s) to Queue__jki_lib_state_machine.vi"("State(s) in Front (\"\")"=w330, "State(s) in (\"\")"=w337) -> ("States Out"=w336:string)  [unwired: 13 in]
          }
          frame "Macro: Exit" {
            # "Exit Macro\n(This is called once, when the VI exits)"
            n113 = Unbundle By Name(w341) -> ("Core.Close Panel on Exit?"=w339:bool)
            n114 = Select(t="UI: Front Panel State >> Close", s=w339, f="") -> (s? t:f=w348:string)
            n115 = call <vilib>:"Add State(s) to Queue__jki_lib_state_machine.vi"("State(s) in Front (\"\")"="Data: Cleanup\nEvents: Unregister\nProcess: Self Terminate", "State(s) in (\"\")"="Process: Sync", "State(s) at Back (\"\")"="Exit") -> ("States Out"=w343:string)  [unwired: 12 in]
            n116 = call <vilib>:"Add State(s) to Queue__jki_lib_state_machine.vi"("State(s) in Front (\"\")"="Action: Close\nMacro: Write UI Config", "State(s) in (\"\")"=w348, "State(s) at Back (\"\")"=w343) -> ("States Out"=w347:string)  [unwired: 12 in]
            n117 = call <vilib>:"Add State(s) to Queue__jki_lib_state_machine.vi"("State(s) in Front (\"\")"=w347, "State(s) in (\"\")"=w352) -> ("States Out"=w351:string)  [unwired: 13 in]
          }
          frame "---------- Process ----------" {
            # "Template Separator\n(You can make a copy of, or modify, this frame)"
            n118 = call <vilib>:"Add State(s) to Queue__jki_lib_state_machine.vi"("State(s) in (\"\")"=w357) -> ("States Out"=w356:string)  [unwired: 14 in]
          }
          frame "Process: Sync" {
            n119 = Unbundle By Name(w365) -> ("Instrument UI"=w361:refnum<class "Instrument UI.Framework-Template.lvclass">)
            n120 = call <vilib>:"WaitOnProcessSync.vi"("error in (no error)"=w360, "SMO"=w361) -> ("error out"=w359:errorcluster, "Don't run?"=w364:bool)  [unwired: 7 in, 1 out]
            n121 = Select(t="Data: Cleanup\nEvents: Unregister\nExit", s=w364, f="") -> (s? t:f=w358:string)
            n122 = call <vilib>:"Add State(s) to Queue__jki_lib_state_machine.vi"("State(s) in Front (\"\")"=w358, "State(s) in (\"\")"=w368) -> ("States Out"=w367:string)  [unwired: 13 in]
          }
          frame "Process: Self Terminate" {
            n123 = Unbundle By Name(w370) -> ("Instrument UI"=w369:refnum<class "Instrument UI.Framework-Template.lvclass">)
            n124 = call <vilib>:"SelfTerminate.vi"("error in (no error)"=w372, "SMO in"=w369) -> ("error out"=w371:errorcluster)  [unwired: 8 in, 1 out]
            n125 = call <vilib>:"Add State(s) to Queue__jki_lib_state_machine.vi"("State(s) in (\"\")"=w375) -> ("States Out"=w374:string)  [unwired: 14 in]
          }
          frame "---------- Events ----------" {
            # "Template Separator\n(You can make a copy of, or modify, this frame)"
            n126 = call <vilib>:"Add State(s) to Queue__jki_lib_state_machine.vi"("State(s) in (\"\")"=w380) -> ("States Out"=w379:string)  [unwired: 14 in]
          }
          frame "Events: Register" {
            # "Expand to add\nmore events"
            # "Base Class Protected Events"
            n127 = Unbundle By Name(w391) -> ("Instrument UI"=w382:refnum<class "Instrument UI.Framework-Template.lvclass">, "Instrument"=w381:refnum<class "Instrument.Framework-Template.lvclass">)
            n128 = call <vilib>:"GetProtectedEvents.vi"("SMO"=w382) -> ("error out"=w385:errorcluster, "SMO Protected Events"=w389:T9)  [unwired: 8 in, 1 out]
            n129 = call <userlib>:"Instrument.GetPublicEvents.vi"("Instrument"=w381) -> ("error out"=w383:errorcluster, "Instrument Public Events"=w384:T10)  [unwired: 8 in, 1 out]
            n130 = register-events(w389, w384) -> (reference out=w390:refnum<event-registration>, error out=w387:errorcluster)  [unwired: 2 in]
            n131 = Merge Errors(w383, w388, w387, w385) -> (w386:errorcluster)
            n132 = call <vilib>:"Add State(s) to Queue__jki_lib_state_machine.vi"("State(s) in (\"\")"=w393) -> ("States Out"=w392:string)  [unwired: 14 in]
          }
          frame "Events: Unregister" {
            n133 = Unregister For Events(event registration refnum=w396, error in=w395) -> (error out=w394:errorcluster)
            n134 = call <vilib>:"Add State(s) to Queue__jki_lib_state_machine.vi"("State(s) in (\"\")"=w399) -> ("States Out"=w398:string)  [unwired: 14 in]
          }
          frame "---------- Configuration ----------" {
            # "Do not put any code in this frame.\n(It is a separator no-op. You can make a copy of this frame to create a new UI frame)"
            n135 = call <vilib>:"Add State(s) to Queue__jki_lib_state_machine.vi"("State(s) in (\"\")"=w404) -> ("States Out"=w403:string)  [unwired: 14 in]
          }
          frame "Configuration: Initialize" {
            # "Do not put any code in this frame.\n(It is a separator no-op. You can make a copy of this frame to create a new UI frame)"
            n136 = Unbundle By Name(w412) -> ("Configuration"=w410:refnum<class "Configuration.lvclass">, "Instrument"=w411:refnum<class "Instrument.Framework-Template.lvclass">)
            n137 = call <vilib>:"GetName.vi"("error in (no error)"=w414, "SMO"=w411) -> ("error out"=w413:errorcluster, "Name"=w415:string)  [unwired: 6 in, 2 out]
            n138 = call <userlib>:"Default Path.vi"("error in (no error)"=w413, "Folder Name [Application Name]"=w415, "Configuration in"=w410) -> ("error out"=w406:errorcluster, "Configuration out"=w409:refnum<class "Configuration.lvclass">)  [unwired: 7 in]
            n139 = call <userlib>:"Write Section.vi"("error in (no error)"=w406, "Section"="UI", "Configuration in"=w409) -> ("error out"=w405:errorcluster, "Configuration out"=w408:refnum<class "Configuration.lvclass">)  [unwired: 7 in]
            n140 = Bundle By Name(cluster=w412, "Configuration"=w408) -> (w416:T6)
            n141 = call <vilib>:"Add State(s) to Queue__jki_lib_state_machine.vi"("State(s) in (\"\")"=w419) -> ("States Out"=w418:string)  [unwired: 14 in]
          }
          frame "Configuration: Write UI Config File" {
            # "Do not put any code in this frame.\n(It is a separator no-op. You can make a copy of this frame to create a new Data frame)"
            n142 = Unbundle By Name(w424) -> ("Configuration"=w421:refnum<class "Configuration.lvclass">, "UI Cluster"=w423:T5)
            n143 = call <userlib>:"Write Configuration.vi"("error in (no error)"=w420, "Variant"=w423, "Configuration in"=w421) -> ("error out"=w422:errorcluster)  [unwired: 7 in, 1 out]
            n144 = call <vilib>:"Add State(s) to Queue__jki_lib_state_machine.vi"("State(s) in (\"\")"=w427) -> ("States Out"=w426:string)  [unwired: 14 in]
          }
          frame "Configuration: Read UI Config File" {
            # "Do not put any code in this frame.\n(It is a separator no-op. You can make a copy of this frame to create a new UI frame)"
            n145 = Unbundle By Name(w430) -> ("UI Cluster"=w433:T5, "Configuration"=w436:refnum<class "Configuration.lvclass">)
            n146 = call <userlib>:"Read Configuration.vi"("INI Fomatted Cluster Type"=w433, "error in (no error)"=w432, "Configuration in"=w436) -> ("error out"=w435:errorcluster, "Configuration"=w434:variant)  [unwired: 6 in, 1 out]
            n147 = Variant To Data(error in=w435, type=w433, Variant=w434) -> (data=w429:T5, error out=w431:errorcluster)
            n148 = Bundle By Name(cluster=w430, "UI Cluster"=w429) -> (w428:T6)
            n149 = call <vilib>:"Add State(s) to Queue__jki_lib_state_machine.vi"("State(s) in (\"\")"=w439) -> ("States Out"=w438:string)  [unwired: 14 in]
          }
          frame "---------- Action ----------" {
            n150 = Unbundle By Name(w442) -> ("Instrument UI"=w440:refnum<class "Instrument UI.Framework-Template.lvclass">)
            n151 = Bundle By Name(cluster=w442, "Instrument UI"=w440) -> (w441:T6)
            n152 = call <vilib>:"Add State(s) to Queue__jki_lib_state_machine.vi"("State(s) in (\"\")"=w446) -> ("States Out"=w445:string)  [unwired: 14 in]
          }
          frame "Action: Notify UI Closed" {
            # "Notify that the UI has been closed"
            n153 = Unbundle By Name(w447) -> ("Instrument UI"=w450:refnum<class "Instrument UI.Framework-Template.lvclass">)
            n154 = call <vilib>:"Hide.vi"("error in (no error)"=w449, "SMO.UI"=w450) -> ("error out"=w448:errorcluster)  [unwired: 8 in, 1 out]
            n155 = call <vilib>:"Add State(s) to Queue__jki_lib_state_machine.vi"("State(s) in (\"\")"=w453) -> ("States Out"=w452:string)  [unwired: 14 in]
          }
          frame "Action: getAll" {
            n156 = Unbundle By Name(w462) -> ("getAll"=w455:T4, "Instrument"=w456:refnum<class "Instrument.Framework-Template.lvclass">)
            n157 = call <userlib>:"getAll.vi"("error in (no error)"=w454, "Instrument in"=w456) -> ("error out"=w461:errorcluster, "getAll"=w457:variant, "Instrument out"=w458:refnum<class "Instrument.Framework-Template.lvclass">)  [unwired: 7 in]
            n158 = call "JSON to LVtype.vim"("type"=w455, "error in (no error)"=w461, "JSON Data in"=w457) -> ("error out"=w460:errorcluster, "Data out"=w459:T4)  [unwired: 7 in]
            n159 = Bundle By Name(cluster=w462, "Instrument"=w458, "getAll"=w459) -> (w463:T6)
            n160 = call <vilib>:"Add State(s) to Queue__jki_lib_state_machine.vi"("State(s) in Front (\"\")"="" ("State(s) in Front (\"\")"), "State(s) in (\"\")"=w467) -> ("States Out"=w466:string)  [unwired: 13 in]
          }
          frame "Action: Open" {
            # "local/remote?"
            n161 = Unbundle By Name(w471) -> ("Instrument"=w469:refnum<class "Instrument.Framework-Template.lvclass">)
            n162 = call-dynamic "Open.vi"("error in (no error)"=w468, "Instrument.Framework-Template in"=w469) -> ("error out"=w474:errorcluster, "Instrument.Framework-Template out"=w470:refnum<class "Instrument.Framework-Template.lvclass">)  [unwired: 8 in]
            n163 = Bundle By Name(cluster=w471, "Instrument"=w470) -> (w472:T6)
            n164 = call <vilib>:"Add State(s) to Queue__jki_lib_state_machine.vi"("State(s) in Front (\"\")"="" ("State(s) in Front (\"\")"), "State(s) in (\"\")"=w477) -> ("States Out"=w476:string)  [unwired: 13 in]
          }
          frame "Action: Close" {
            n165 = Unbundle By Name(w479) -> ("Instrument"=w482:refnum<class "Instrument.Framework-Template.lvclass">)
            n166 = call-dynamic "Close.vi"("error in (no error)"=w480, "Instrument.Framework-Template in"=w482) -> ("error out"=w484:errorcluster, "Instrument.Framework-Template out"=w478:refnum<class "Instrument.Framework-Template.lvclass">)  [unwired: 8 in]
            n167 = Bundle By Name(cluster=w479, "Instrument"=w478) -> (w481:T6)
            n168 = call <vilib>:"Add State(s) to Queue__jki_lib_state_machine.vi"("State(s) in Front (\"\")"="" ("State(s) in Front (\"\")"), "State(s) in (\"\")"=w487) -> ("States Out"=w486:string)  [unwired: 13 in]
          }
        }
      }
    }
    frame Error {
    }
  }
  n169 = call-parent "Process.vi"("error in"=w5, "Instrument UI in"=w4) -> ("error out"=w2:errorcluster, "Instrument UI out"=→"Instrument UI.Framework-Template out":refnum<class "Instrument UI.Framework-Template.lvclass">)  [unwired: 8 in]
  n170 = Merge Errors(w2, w1) -> (→"error out":errorcluster)
